vi "Redirect.vi"(6 "LabVIEW Web Service Request":refnum<class "Web Request.lvclass">) -> (1 "query string":string)   [LabVIEW 2020]
doc: "Redirect callback VI: when we'll call the authentication endpoint, it will call us back at the https://localhost:8001/OAuth/Redirect.URL that executes this VI."
uses:
  <vilib>/wsapi/Web Request.lvclass
  subVIs/globals.vi
  Netatmo-WeatherStation.lvlib
panel:
  out "appended array":string[][](array[string])
  # "Each additional control wired to the connector pane will be available as an input in the URL. To include an indicator in terminal-mode output (the default setting), it must also be wired to the connector pane."
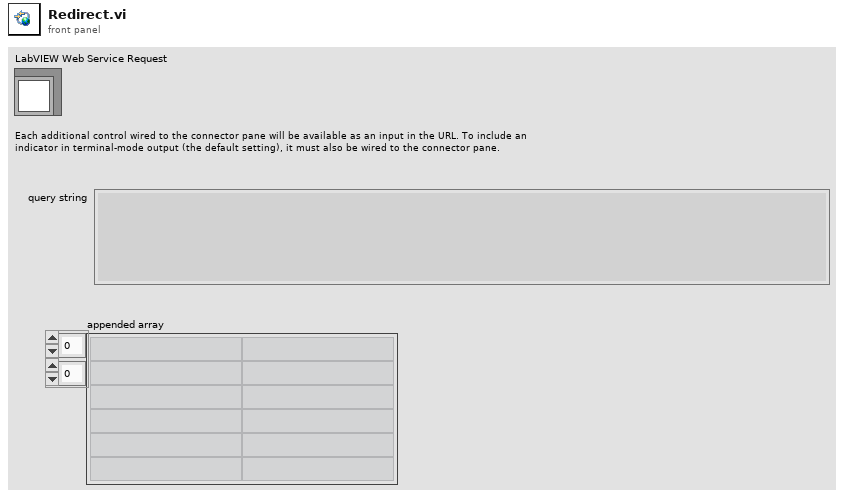
[diagram p1: front panel]
types:
  T1 = cluster{"Redirect Data":refnum<user-event>, "Redirect Error":refnum<user-event>}
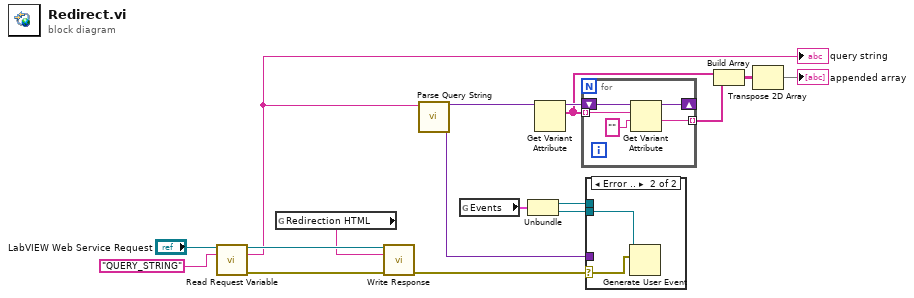
[diagram p0: block diagram]
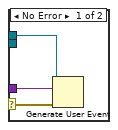
[diagram p2: hidden frame]
diagram:
  n1 = call <vilib>:"Read Request Variable.vi"("LabVIEW Web Service Request"="LabVIEW Web Service Request", "variable name"="QUERY_STRING") -> ("LabVIEW Web Service Request out"=w14:refnum<class "Web Request.lvclass">, "value"=w12:string, "error out"=w13:errorcluster)  [unwired: 11 in]
  "query string" <- w12
  n2 = global read "globals.vi" "Redirection HTML"() -> (w5:string)
  n3 = call <vilib>:"Write Response.vi"("LabVIEW Web Service Request"=w14, "response string"=w5, "error in (no error)"=w13) -> ("error out"=w4:errorcluster)  [unwired: 11 in, 1 out]
  n4 = call "Parse Query String.vi"("query string"=w12) -> ("Variant"=w6:variant)  [unwired: 10 in]
  n5 = global read "globals.vi" "Events"() -> (w3:T1)
  n6 = Unbundle(w3) -> ("Redirect Data"=w2:refnum<user-event>, "Redirect Error"=w1:refnum<user-event>)
  n7 = Get Variant Attribute(Variant=w6) -> (duplicate Variant=w11:variant, names=w9:string[])  [unwired: 3 in, 2 out]
  n8 = for {
    shift-right: [w20] -> _
    shift-left: w11 -> [w21]
    tunnel: w9 -> [w19] mode=indexing
    tunnel: [w17] -> w10 mode=indexing
    n9 = Get Variant Attribute(Variant=w21, name=w19, default value (empty Variant)="") -> (duplicate Variant=w20:variant, value=w17:string)  [unwired: 1 in, 2 out]
  }
  n10 = case shown="Error .." w4 {
    selector: w4 -> [w22 w25]
    tunnel: w6 -> [w24 _]
    tunnel: w2 -> [w23 _]
    tunnel: w1 -> [_ w26]
    frame No Error {
      n11 = Generate User Event(user event=w23, event data cluster=w24, error in=w22) -> ()  [unwired: 1 in, 2 out]
    }
    frame Error {
      n12 = Generate User Event(user event=w26, event data cluster=w25) -> ()  [unwired: 2 in, 2 out]
    }
  }
  n13 = Build Array(w9, w10) -> (w8:string[][])
  n14 = Transpose 2D Array(2D array=w8) -> (transposed array=→"appended array":string[][])
